vi "UI 1.vi"(8 "error in (no error)":errorcluster, 11 "Event Refs":T1) -> (0 "error out":errorcluster)   [LabVIEW 2010, in "UI 1.lvlib"]
uses:
  UI 1.lvlib
  Launcher/Launcher.lvlib
  Error Handler/Error Handler.lvlib
  Module/User Event Message Enum.ctl
  Module/Template Module.lvlib
  Module/User Event Message Cluster.ctl
  Error Handler/User Event Message Enum.ctl
  Error Handler/User Event Message Cluster.ctl
  Launcher/Event Message Cluster.ctl
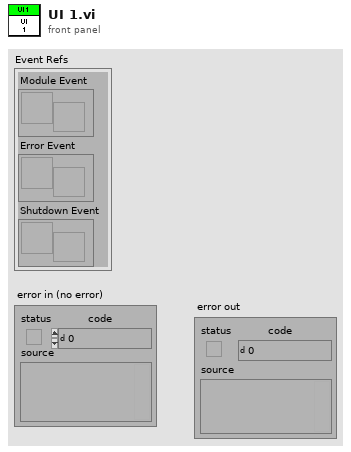
[diagram p1: front panel]
types:
  T1 = typedef "Launcher.lvlib/Event Message Cluster.ctl" = cluster{"Module Event":refnum<user-event>, "Error Event":refnum<user-event>, "Shutdown Event":refnum<user-event>}
  T2 = typedef "Template Module.lvlib/User Event Message Enum.ctl" = enum16{"Event 1"}
  T3 = typedef "Error Handler.lvlib/User Event Message Enum.ctl" = enum16{"Event 1"}
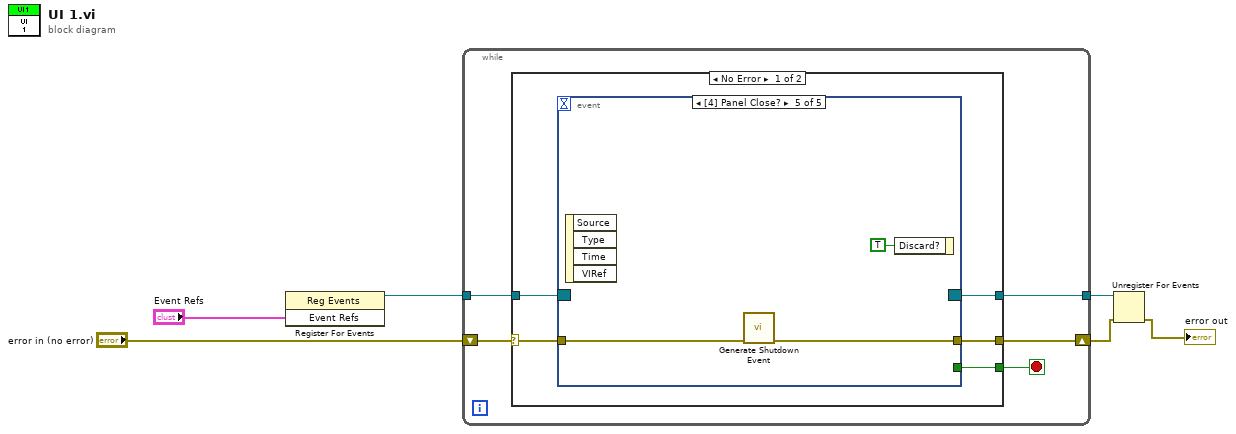
[diagram p0: block diagram]
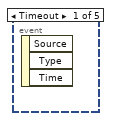
[diagram p2: hidden frame]
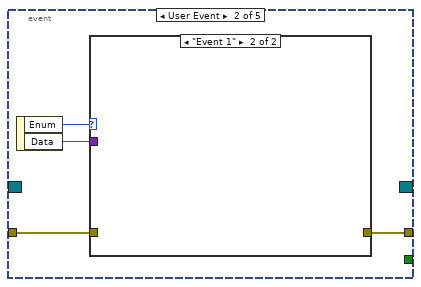
[diagram p3: hidden frame]
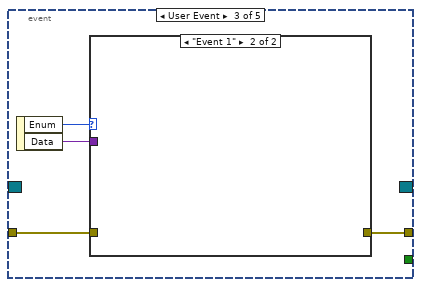
[diagram p5: hidden frame]
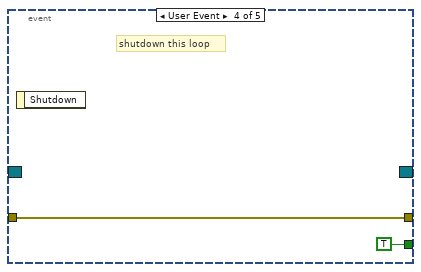
[diagram p7: hidden frame]
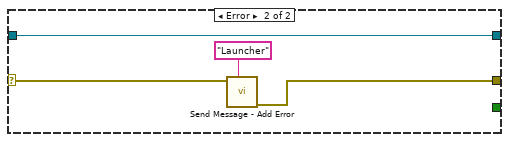
[diagram p8: hidden frame]
diagram:
  n1 = register-events("Event Refs") -> (reference out=w6:refnum<event-registration>)  [unwired: 2 in, 1 out]
  n2 = while {
    shift-right: [w8] -> w4
    shift-left: "error in (no error)" -> [w11]
    tunnel: w6 -> [w10]
    tunnel: [w9] -> w5
    stop <- w7 stop-if-true
    n3 = case shown="No Error" w11 {
      selector: w11 -> [w14 w35]
      tunnel: w10 -> [w16 w33]
      tunnel: [w15 w33] -> w9
      tunnel: [w13 w34] -> w8
      tunnel: [w12 _] -> w7
      frame No Error {
        n4 = event shown="[4] Panel Close?" {
          selector: w16 -> [_ _ _ _ _]
          dyn-events: [_ _ _ _ _] -> w15
          timeout: _ -> [_ _ _ _ _]
          tunnel: w14 -> [_ w19 w24 w27 w30]
          tunnel: [_ w18 w23 w27 w29] -> w13
          tunnel: [_ _ _ TRUE _] -> w12
          event Timeout {
            n5 = event-data() -> ()  [unwired: 1 in, 3 out]
          }
          event User Event {
            n6 = event-data() -> ("Enum"=w20:T2, "Data"=w17:variant)  [unwired: 1 in]
            n7 = case shown="\"Event 1\"" w20 {
              tunnel: w19 -> [w21 _]
              tunnel: [w21 _] -> w18
              tunnel: w17 -> [_ _]
              frame Default {
              }
              frame "Event 1" {
              }
            }
          }
          event User Event {
            n8 = event-data() -> ("Enum"=w25:T3, "Data"=w22:variant)  [unwired: 1 in]
            n9 = case shown="\"Event 1\"" w25 {
              tunnel: w24 -> [w26 _]
              tunnel: [w26 _] -> w23
              tunnel: w22 -> [_ _]
              frame Default {
              }
              frame "Event 1" {
              }
            }
          }
          event User Event {
            # "shutdown this loop"
            n10 = event-data() -> ()  [unwired: 1 in, 1 out]
          }
          event Panel Close? {
            n11 = event-data() -> ()  [unwired: 1 in, 4 out]
            n12 = call "Generate Shutdown Event.vi"("error in (no error)"=w30) -> ("error out"=w29:errorcluster)  [unwired: 10 in]
            n13 = event-data("Discard?"=TRUE) -> ()  [unwired: 1 in, 1 out]
          }
        }
      }
      frame Error {
        n14 = call "Send Message - Add Error.vi"("Source"="Launcher", "Error to Handle"=w35) -> ("error out"=w34:errorcluster)  [unwired: 9 in]
      }
    }
  }
  n15 = Unregister For Events(event registration refnum=w5, error in=w4) -> (error out=→"error out":errorcluster)
